vi "Main.vi"() -> ()   [LabVIEW 2014, in "6. Reusing Components Dynamically.lvlib"]
doc: "We dynamically generate a grid of Number Widgets from example \"5. Creating a User-Defined Signal\". We also dynamically connect the widgets' signals to a callback such that updating one Number Widget will auto-update all Number Widgets that come after it.\n\n\n<b>Showcase</b>\n- Reusing (multiple instances of) a user-defined, subclassed widget\n- Dynamically composing a GUI, based on user input\n- Dynamically setting up event-driven communications between widgets, without (explicitly) creating an Event structure.\n\n\nCopyright (c) 2019 Sze Howe Koh.\nThis code is licensed under the MIT license."
uses:
  6. Reusing Components Dynamically.lvlib
  Number Widget/Number Widget.lvclass
  <vilib>/addons/LQ/LQ Core/LQCoreEngine/LQCoreEngine.lvclass
  <vilib>/addons/LQ/Qt Widgets/QWidget/QWidget.lvclass
  <vilib>/addons/LQ/Qt Widgets/QGridLayout/QGridLayout.lvclass
panel:
  in  "Stop Button":bool
  in  "No. of Columns":i32=3 min=1
  in  "No. of Rows":i32=2 min=1
  in  "Create Grid Button":bool
  # "Prerequisite knowledge/experience\n- Example 3c. Connecting a Signal to a LabVIEW Callback\n- Example 5. Creating a User-Defined Signal\n\n\nDescription\nWe dynamically generate a grid of Number Widgets from example 5. Creating a User-Defined Signal.\nWe also dynamically connect the widgets' signals to a callback such that updating one Number\nWidget will auto-update all Number Widgets that come after it.\n\n\nInstructions\n1. Run this VI and click \"Create Grid\".\n2. Drag the sliders of different Number Widgets, and observe the reaction of other Number Widgets.\n3. Enter a different number of rows and columns, and click \"Create Grid\" again.\n\n\nShowcase\n- Reusing (multiple instances of) a user-defined, subclassed widget\n- Dynamically composing a GUI, based on user input\n- Dynamically setting up event-driven communications between widgets, without (explicitly) creating\n    an Event structure."
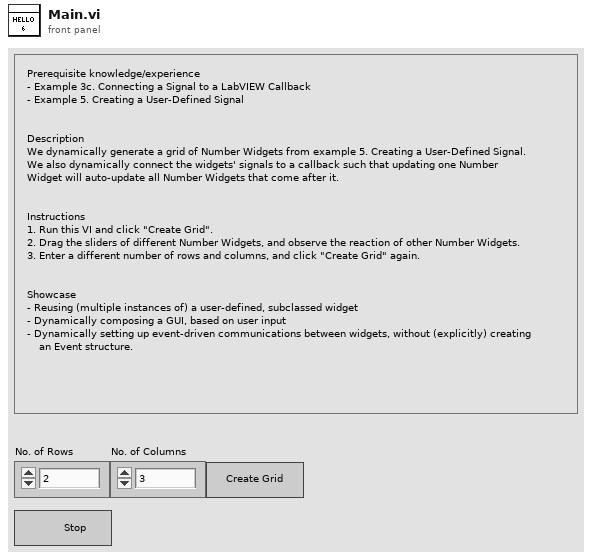
[diagram p1: front panel]
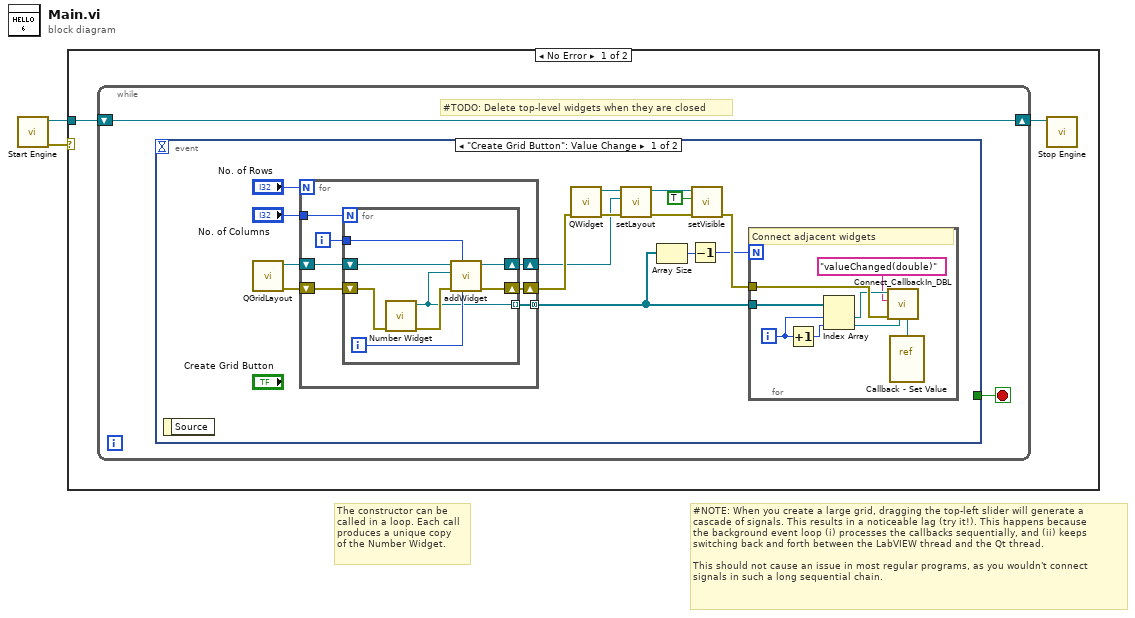
[diagram p0: block diagram]
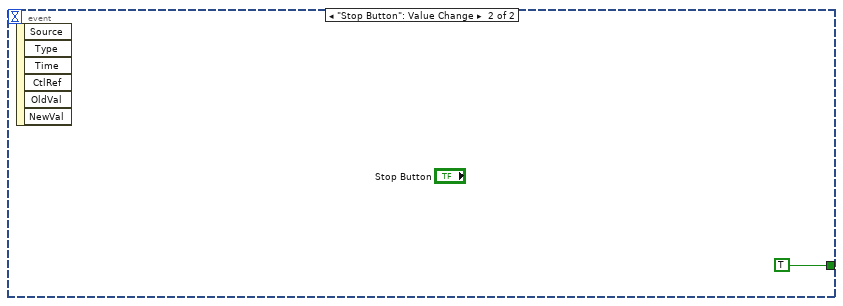
[diagram p2: hidden frame]
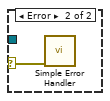
[diagram p3: hidden frame]
diagram:
  # "The constructor can be\ncalled in a loop. Each call\nproduces a unique copy\nof the Number Widget."
  # "#NOTE: When you create a large grid, dragging the top-left slider will generate a\ncascade of signals. This results in a noticeable lag (try it!). This happens because\nthe background event loop (i) processes the callbacks sequentially, and (ii) keeps\nswitching back and forth between the LabVIEW thread and the Qt thread.\n\nThis should not cause an issue in most regular programs, as you wouldn't connect\nsignals in such a long sequential chain."
  n1 = call <vilib>:"Start Engine.vi"() -> ("Error Out"=w2:errorcluster, "New Engine"=w1:refnum<class "LQCoreEngine.lvclass">)  [unwired: 10 in]
  n2 = case shown="No Error" w2 {
    selector: w2 -> [_ w46]
    tunnel: w1 -> [w4 _]
    frame No Error {
      n3 = while {
        shift-right: [w6] -> w3
        shift-left: w4 -> [w6]
        stop <- w5 stop-if-true
        # "#TODO: Delete top-level widgets when they are closed"
        n4 = event shown="[0] \"Create Grid Button\": Value Change" {
          selector: _ -> [_ _]
          dyn-events: _ -> [_ _]
          timeout: _ -> [_ _]
          tunnel: [_ TRUE] -> w5
          event "Create Grid Button": Value Change {
            n5 = event-data() -> ()  [unwired: 1 in, 1 out]
            n6 = call <vilib>:"QGridLayout.vi"() -> ("Error Out"=w17:errorcluster, "New QGridLayout"=w18:refnum<class "QGridLayout.lvclass">)  [unwired: 10 in]
            n7 = for {
              N: "No. of Rows" -> [_]
              tunnel: "No. of Columns" -> [w36]
              shift-right: [w33] -> w11
              shift-left: w18 -> [w35]
              shift-right: [w31] -> w14
              shift-left: w17 -> [w32]
              tunnel: [w30] -> w7 mode=concatenating
              i -> [w34]
              n8 = for {
                N: w36 -> [_]
                shift-right: [w39] -> w33
                shift-left: w35 -> [w43]
                tunnel: w34 -> [w37]
                shift-right: [w41] -> w31
                shift-left: w32 -> [w40]
                tunnel: [w38] -> w30 mode=indexing
                i -> [w42]
                n9 = call "Number Widget.vi"("Error In"=w40) -> ("Error Out"=w44:errorcluster, "New Number Widget"=w38:refnum<class "Number Widget.lvclass">)  [unwired: 9 in]
                n10 = call <vilib>:"addWidget.vi"("column"=w42, "row"=w37, "Error In"=w44, "widget"=w38, "QGridLayout In"=w43) -> ("Error Out"=w41:errorcluster, "QGridLayout Out"=w39:refnum<class "QGridLayout.lvclass">)  [unwired: 5 in]
              }
            }
            n11 = call <vilib>:"QWidget.vi"("Error In"=w14) -> ("Error Out"=w12:errorcluster, "New QWidget"=w13:refnum<class "QWidget.lvclass">)  [unwired: 9 in]
            n12 = call <vilib>:"setLayout.vi"("Error In"=w12, "layout"=w11, "QWidget In"=w13) -> ("Error Out"=w10:errorcluster, "QWidget Out"=w9:refnum<class "QWidget.lvclass">)  [unwired: 7 in]
            n13 = Array Size(array=w7) -> (size(s)=w16:i32)
            n14 = Decrement(x=w16) -> (x-1=w15:i32)
            n15 = call <vilib>:"setVisible.vi"("Error In"=w10, "visible"=TRUE, "QWidget In"=w9) -> ("Error Out"=w21:errorcluster)  [unwired: 7 in, 1 out]
            n16 = for {
              N: w15 -> [_]
              tunnel: w7 -> [w28]
              tunnel: w21 -> [w29]
              i -> [w25]
              # "Connect adjacent widgets"
              n17 = Increment(x=w25) -> (x+1=w24:i32)
              n18 = Index Array(array=w28, index #1=w25, index #2=w24) -> (element #1=w27:refnum<class "Number Widget.lvclass">, element #2=w26:refnum<class "Number Widget.lvclass">)
              n19 = vi-ref "Callback - Set Value.vi"() -> (w23:refnum<vi>)
              n20 = call <vilib>:"Connect_CallbackIn_DBL.vi"("Slot VI"=w23, "Receiver"=w26, "Error In"=w29, "Signal"="valueChanged(double)", "Sender In"=w27) -> ()  [unwired: 5 in, 2 out]
            }
          }
          event "Stop Button": Value Change {
            n21 = event-data() -> ()  [unwired: 1 in, 6 out]
          }
        }
      }
      n22 = call <vilib>:"Stop Engine.vi"("LQCoreEngine"=w3) -> ()  [unwired: 10 in, 1 out]
    }
    frame Error {
      n23 = call <vilib>:"Simple Error Handler.vi"("error in (no error)"=w46) -> ()  [unwired: 4 in, 5 out]
    }
  }
